vi "Heartbeat Monitor VI.vi"() -> ()   [LabVIEW 2015]
uses:
  <vilib>/express/express analysis/Spectral/Block/exnSpectralBlock spectral measurements power poly.vi
  <vilib>/express/express analysis/Spectral/Block/exnSpectralBlock spectral measurements power DDT.vi
  <vilib>/express/express analysis/Spectral/XNode/ExpressSpectralMeasurementsBlockNode.xnode
panel:
  in  "Starting Parameters":cluster{"Rate":dbl, "Time":dbl}={"Rate"=10000.0, "Time"=10.0}
  out "df":dbl
  out "Frequency Plot":dynamicdata(graph) caption="Section"
  out "Heart Beat":dbl
  in  "STOP":bool
  out "Filtered Time Plot":dynamicdata(graph)=[{"t0"=timestamp(3532474759.3784313 s since 1904-01-01), "dt"=9.999999999999999e-05, "Y"=array[100000 elements], "attributes"=variant("NI_ChannelName"=variant(string "Voltage (Filtered)"), "NI_OriginalChannelName"=variant(string "Voltage"), "NI_UnitDescription"=variant(string "Volts"))}] caption="Filtered Signal"
  out "data":dynamicdata(graph)=[{"t0"=timestamp(3532474759.3784313 s since 1904-01-01), "dt"=9.999999999999999e-05, "Y"=array[100000 elements], "attributes"=variant("NI_ChannelName"=variant(string "Voltage"), "NI_UnitDescription"=variant(string "Volts"))}] caption="Unfilitered Time Plot"
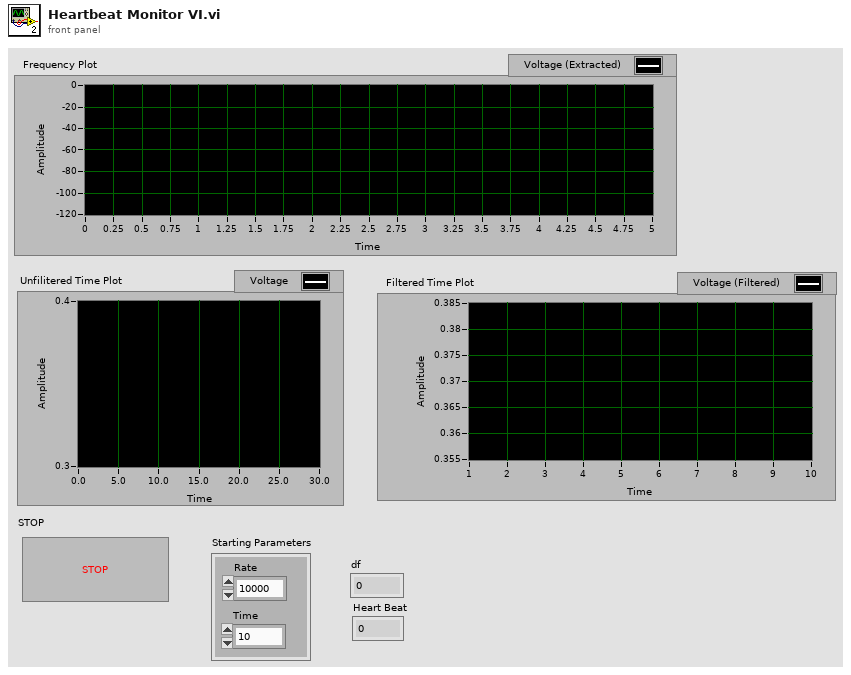
[diagram p1: front panel]
types:
  T1 = cluster{"averaging mode":u16, "weighting mode":u16, "number of averages":u32}
  T2 = cluster{"dB On (F)":bool, "unwrap phase (F)":bool, "convert to degree (F)":bool}
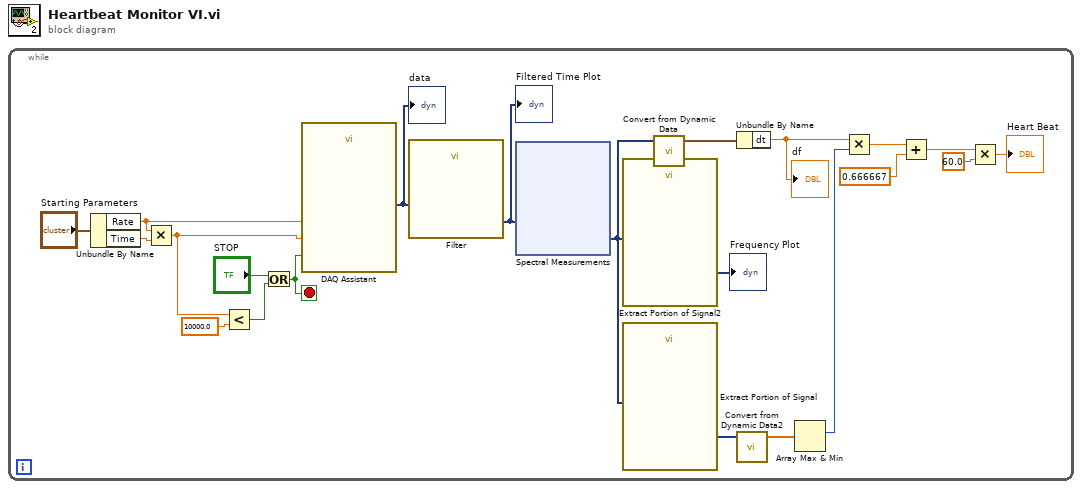
[diagram p0: block diagram]
diagram:
  n1 = while {
    stop <- w20 stop-if-true
    n2 = Unbundle By Name("Starting Parameters") -> ("Rate"=w2:dbl, "Time"=w1:dbl)
    n3 = Multiply(x=w2, y=w1) -> (x*y=w17:dbl)
    n4 = Less?(x=w17, y=10000.0) -> (x < y?=w21:bool)
    n5 = Or(x="STOP", y=w21) -> (x .or. y?=w20:bool)
    n6 = call "DAQ Assistant"("rate"=w2, "number of samples"=w17, "stop (T)"=w20) -> ("data"=w19:dynamicdata)  [unwired: 14 in, 2 out]
    "data" <- w19
    n7 = call "Filter"("Signal"=w19) -> ("Filtered Signal"=w4:dynamicdata)  [unwired: 9 in, 1 out]
    "Filtered Time Plot" <- w4
    n8 = xnode "Spectral Measurements"("Signals"=w4) -> ("Power Spectrum"=w7:dynamicdata)  [unwired: 1 in, 1 out]
    n9 = call "Extract Portion of Signal2"("Signals"=w7) -> ("Section"=→"Frequency Plot":dynamicdata)  [unwired: 9 in, 1 out]
    n10 = call "Extract Portion of Signal"("Signals"=w7) -> ("Section"=w12:dynamicdata)  [unwired: 9 in, 1 out]
    n11 = call "Convert from Dynamic Data"("Dynamic Data Type"=w7) -> ("Waveform"=w6:waveform(dbl))  [unwired: 3 in]
    n12 = Unbundle By Name(w6) -> ("dt"=w5:dbl)
    "df" <- w5
    n13 = call "Convert from Dynamic Data2"("Dynamic Data Type"=w12) -> ("Array"=w14:dbl[])  [unwired: 3 in]
    n14 = Array Max & Min(array=w14) -> (max index (indices)=w8:i32)  [unwired: 3 out]
    n15 = Multiply(x=w5, y=w8) -> (x*y=w11:dbl)
    n16 = Add(x=w11, y=0.666667) -> (x+y=w9:dbl)
    n17 = Multiply(x=w9, y=60.0) -> (x*y=→"Heart Beat":dbl)
  }
